vi "DSF Transfer Group.Separate Inline and Async.vi"(8 "error in (no error)":errorcluster, 11 "Transfer Groups":refnum<class "Transfer Group.lvclass">[](array[class])) -> (0 "error out":errorcluster, 2 "Async Transfer Groups":refnum<class "Transfer Group.lvclass">[](array[class]), 3 "Inline Transfer Groups":refnum<class "Transfer Group.lvclass">[](array[class]))   [LabVIEW 2017, in "DSF.Engine.lvlib" / "Transfer Group.lvclass"]
uses:
  Transfer Group.lvclass
  Transfer Group.lvclass/Transfer Group.ctl
  Timing/Timing.lvclass/Timing.ctl
  Timing/Timing.lvclass
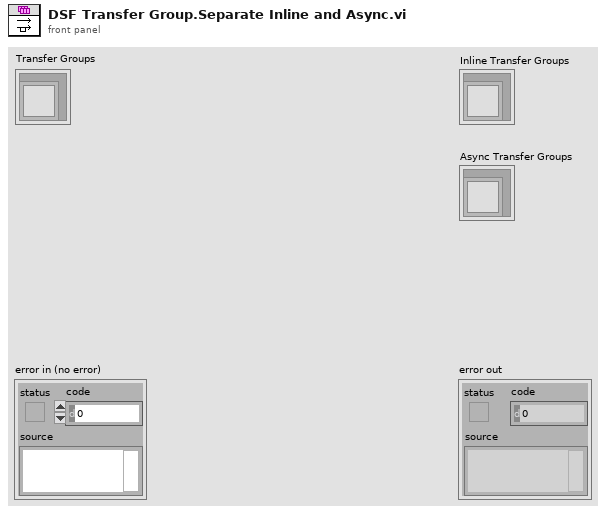
[diagram p1: front panel]
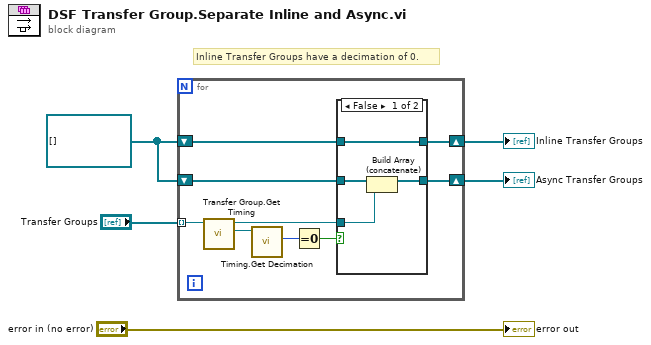
[diagram p0: block diagram]
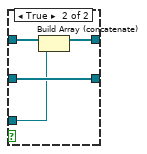
[diagram p2: hidden frame]
diagram:
  w3 = refnum<class "Transfer Group.lvclass">[] [] ("Transfer Groups")
  # "Inline Transfer Groups have a decimation of 0."
  n1 = for {
    tunnel: "Transfer Groups" -> [w14] mode=indexing
    shift-right: [w7] -> w2
    shift-left: w3 -> [w11]
    shift-right: [w6] -> w1
    shift-left: w3 -> [w8]
    n2 = call "Transfer Group.Get Timing.vi"("Transfer Group in"=w14) -> ("Timing"=w13:refnum<class "Timing.lvclass">, "Transfer Group out"=w9:refnum<class "Transfer Group.lvclass">)  [unwired: 9 in]
    n3 = call "Timing.Get Decimation.vi"("Timing in"=w13) -> ("Decimation"=w12:u64)  [unwired: 9 in, 1 out]
    n4 = Equal To 0?(x=w12) -> (x = 0?=w10:bool)
    n5 = case shown="False" w10 {
      tunnel: w11 -> [w18 w21]
      tunnel: w9 -> [w17 w19]
      tunnel: w8 -> [w16 w22]
      tunnel: [w18 w20] -> w7
      tunnel: [w15 w22] -> w6
      frame False {
        n6 = Build Array (concatenate)(w16, w17) -> (w15:refnum<class "Transfer Group.lvclass">[])
      }
      frame True {
        n7 = Build Array (concatenate)(w21, w19) -> (w20:refnum<class "Transfer Group.lvclass">[])
      }
    }
  }
  "Inline Transfer Groups" <- w2
  "Async Transfer Groups" <- w1
  "error out" <- "error in (no error)"
